vi "niFpgaFFTOutsideSCTLCore.vi"(0 "real data in":fxp<+/-,16,1> format="%#.16g", 1 "reset":bool, 5 "imaginary data in":fxp<+/-,16,1> format="%#.16g") -> (3 "data index":u16, 4 "real data out":fxp<+/-,16,6> format="%.12g", 6 "imaginary data out":fxp<+/-,16,6> format="%.12g", 8 "output valid":bool)   [LabVIEW 2017]
uses:
  <vilib>/rvi/LocalResourceManager/LocalResourceManager.xnode
  <vilib>/rvi/FXPMathLib/basic elements/FxpDiscreteDelay/XNode/nifxpmath_DiscreteDelay.xnode
  <vilib>/Platform/TimedLoop/XDataNode/XDataNode.xnode
  <vilib>/Platform/TimedLoop/XDataNode/nitl_modes.ctl
  <vilib>/Platform/TimedLoop/XDataNode/XDNodeRunTimeDep.lvlib
  <vilib>/Platform/TimedLoop/XDataNode/wakeup.ctl
  <vilib>/Platform/TimedLoop/XDataNode/timing_clust.ctl
  <vilib>/rvi/DataTransferAndStorage/Container/XNode/niFpgaContainer.xnode
  <vilib>/rvi/Memory/Memory_Emulation/niFpgaMemoryEmulationRefIn.vi
  <vilib>/rvi/DataTransferAndStorage/Container/Common/niFpgaContainerGetUniqueNameForEmu.vi
  <vilib>/rvi/DataTransferAndStorage/Container/Common/niFpgaContainerSetEmuInfo.vi
  <vilib>/rvi/eio/common/nirviEmuReportErrorAndStop.vi
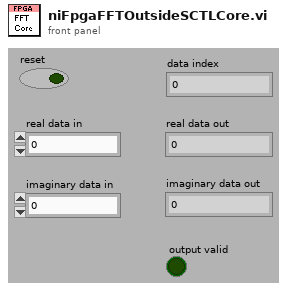
[diagram p1: front panel]
types:
  T1 = typedef "XDNodeRunTimeDep.lvlib/timing_clust.ctl" = cluster{"Expected End [f-1]":u64, "Actual End [f-1]":u64, "Finished Late? [f-1]":bool, "Expected End [i-1]":u64, "Actual End [i-1]":u64, "Finished Late? [i-1]":bool, "Expected Start [i]":u64, "Actual Start [i]":u64, "Expected Start [f]":u64, "Actual Start [f]":u64, "Source Name":string, "Structure Name":string, "Period":i64, "Deadline":i64, "Offset":i64, "Start":i64, "Priority":i32, "Timeout":i32, "Mode":T2, "Wakeup Reason":T3, "Error":errorcluster, "Source Type":string, "Secondary Source Type":string, "Global End Time":u64, "Global Start Time":u64, "Frame Duration":u64, "Iteration Duration":u64, "Assigned CPU":i32, "I/O Scan Engine Mode":u32}
  T2 = typedef "XDNodeRunTimeDep.lvlib/nitl_modes.ctl" = enum32{"No Change", "Process missed periods, maintain original phase", "Discard missed periods, maintain original phase", "Process missed periods, ignore original phase", "Discard missed periods, ignore original phase"}
  T3 = typedef "XDNodeRunTimeDep.lvlib/wakeup.ctl" = enum32{"Normal", "Aborted", "Asynchronous wakeup", "Timing source error", "Timed loop error", "Timeout"}
  T4 = cluster{"N/2-1":u16, "(N/2)*K + 1":u16, "N-1":u16, "total latency":u16, "K - 1":u8, "K - 16":i8, "K - 17":i8}
  T5 = cluster{"Real":fxp<+/-,16,1>, "Imaginary":fxp<+/-,16,1>}
  T6 = typedef "niFPGA FFT Outside SCTL Control Signals.ctl" = cluster{"switch":bool, "twiddle address":u16, "stage":u8, "io read address":u16, "io block 1?":bool, "trans write":bool, "io write address":u16, "update outputs":bool, "use transfer":bool, "io mem a?":bool, "io write":bool, "trans read address":u16}
  T7 = cluster{"addr":u16, "enable":bool, "data":cluster{"Real":fxp<+/-,16,1>, "Imaginary":fxp<+/-,16,1>}}
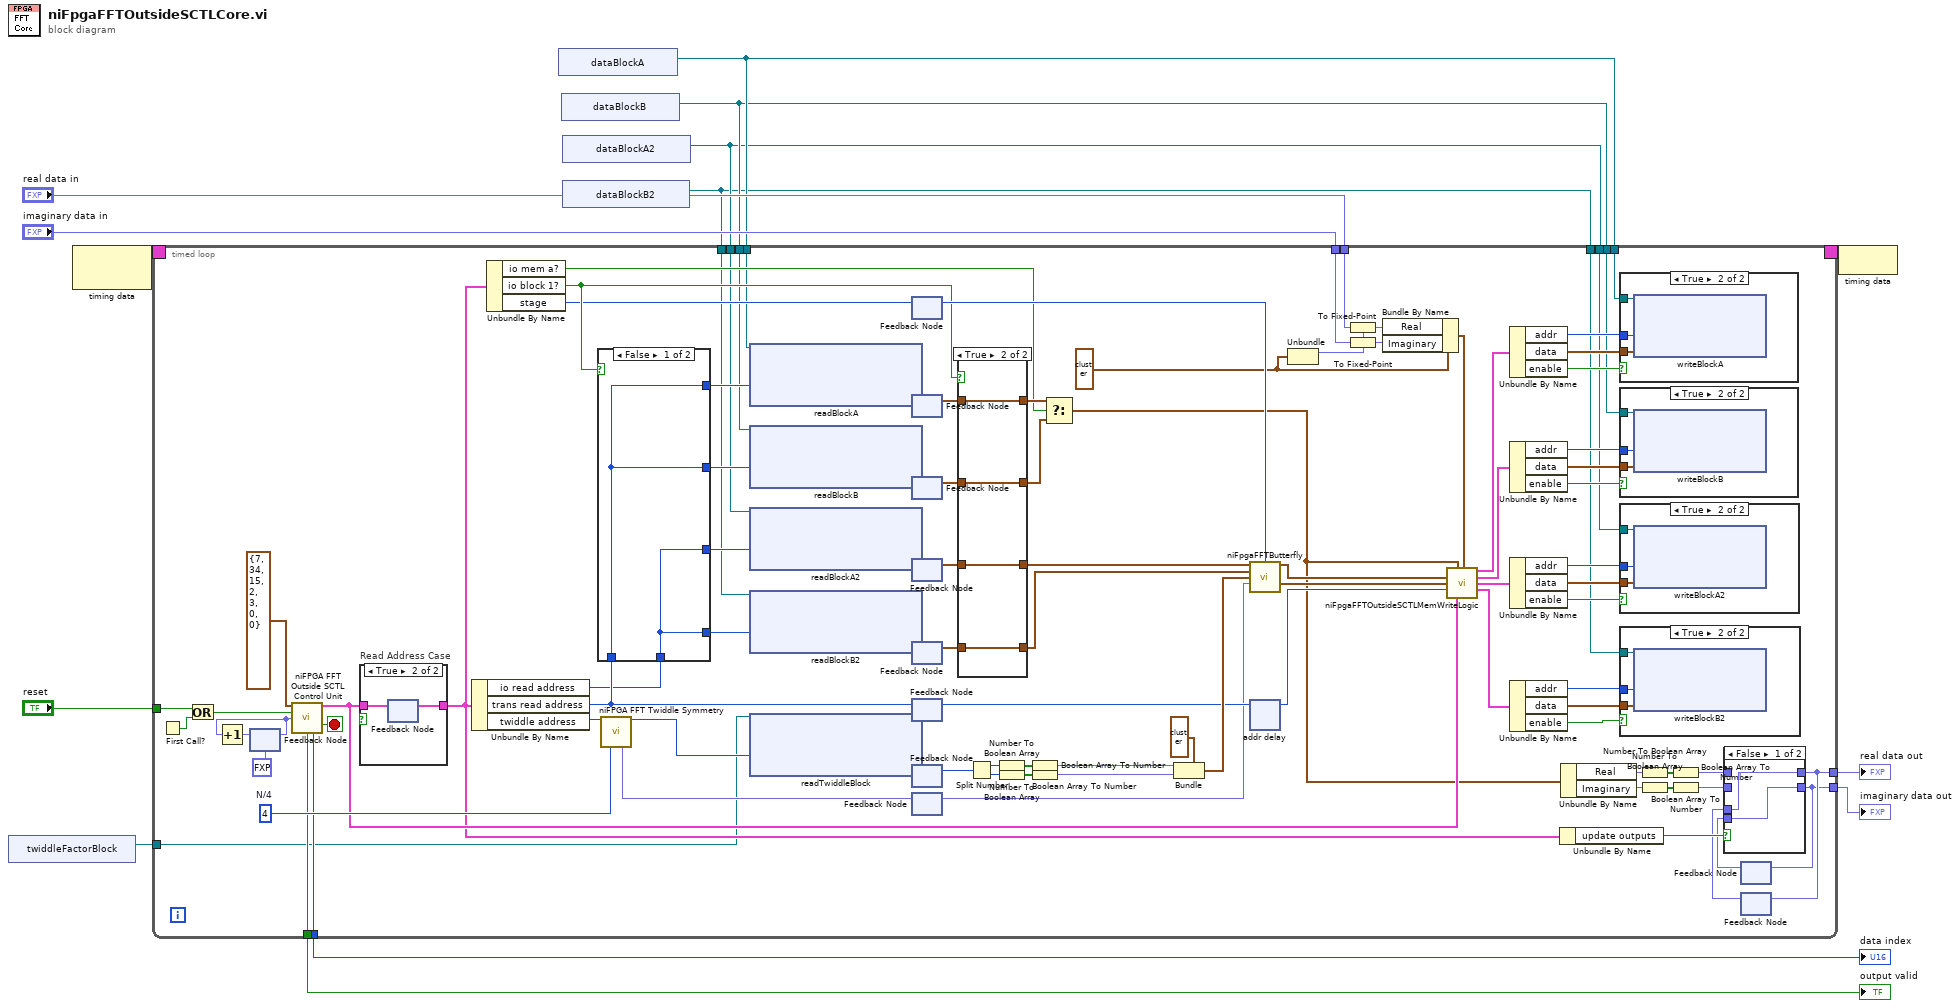
[diagram p0: block diagram]
diagram:
  n1 = xnode "twiddleFactorBlock"() -> ("Memory Out"=w5:refnum<k21>)
  n2 = node-c288() -> (w14:T1)  [unwired: 1 in]
  n3 = xnode "dataBlockA"() -> ("Memory Out"=w4:refnum<k21>)
  n4 = xnode "dataBlockB"() -> ("Memory Out"=w3:refnum<k21>)
  n5 = xnode "dataBlockA2"() -> ("Memory Out"=w2:refnum<k21>)
  n6 = xnode "dataBlockB2"() -> ("Memory Out"=w1:refnum<k21>)
  n7 = timed-loop {
    timing: w14 -> [_]
    timing-out: [_] -> w13
    tunnel: [w53] -> w12
    tunnel: "real data in" -> [w59]
    tunnel: "imaginary data in" -> [w58]
    tunnel: [w55] -> w9
    tunnel: [w54] -> w8
    tunnel: [w52] -> w7
    tunnel: "reset" -> [w30]
    tunnel: w5 -> [w23]
    tunnel: w4 -> [w22]
    tunnel: w3 -> [w21]
    tunnel: w4 -> [w20]
    tunnel: w3 -> [w19]
    tunnel: w2 -> [w18]
    tunnel: w1 -> [w17]
    tunnel: w2 -> [w16]
    tunnel: w1 -> [w15]
    stop <- w50 stop-if-true
    w81 = u16 4  # N/4
    w38 = T5 {"Real"=0.0, "Imaginary"=0.0} ("internalComplexType")
    n8 = First Call?() -> (First Call?: T/F=w32:bool)
    n9 = Or(x=w30, y=w32) -> (x .or. y?=w31:bool)
    n10 = feedback #1(fxp<+,3,3> 0.0) -> (w48:fxp<+,3,3>)
    n11 = Increment(x=w48) -> (x+1=w49:fxp<+,3,3>)
    n12 = feedback-in #1(w49) -> ()
    n13 = call <vilib>:"niFPGA FFT Outside SCTL Control Unit.vi"("Execution Constants"=T4 {"N/2-1"=7, "(N/2)*K + 1"=34, "N-1"=15, "total latency"=2, "K - 1"=3, "K - 16"=0, "K - 17"=0}, "reset"=w31, "iteration"=w48) -> ("control signals out"=w28:T6, "stop"=w50:bool, "output valid"=w52:bool, "data index"=w53:u16)  [unwired: 9 in]
    n14 = case "Read Address Case" shown="True" {
      selector: _ -> [_ _]
      tunnel: w28 -> [w112 w114]
      tunnel: [w112 w113] -> w27
      frame False {
      }
      frame True {
        n15 = feedback-in #2(w114) -> ()
        n16 = feedback #2() -> (w113:T6)  [unwired: 1 in]
      }
    }
    n17 = Unbundle By Name(w27) -> ("io read address"=w64:u16, "trans read address"=w101:u16, "twiddle address"=w33:u16)
    n18 = Unbundle By Name(w27) -> ("io mem a?"=w41:bool, "io block 1?"=w40:bool, "stage"=w29:u8)
    n19 = case shown="False" w40 {
      tunnel: [w127 w130] -> w73
      tunnel: w101 -> [w128 w130]
      tunnel: [w127 w130] -> w72
      tunnel: [w128 w129] -> w71
      tunnel: [w128 w129] -> w70
      tunnel: w64 -> [w127 w129]
      frame False {
      }
      frame True {
      }
    }
    n20 = call <vilib>:"niFPGA FFT Twiddle Symmetry.vi"("twiddle index"=w33, "N/4"=w81) -> ("modified twiddle index"=w37:u16, "flag"=w36:fxp<+,2,2>)  [unwired: 12 in]
    n21 = xnode ("readBlockA")("Address"=w71, "Memory In"=w22) -> ("Data"=w45:T5)  [unwired: 1 out]
    n22 = xnode ("readBlockB")("Address"=w70, "Memory In"=w21) -> ("Data"=w42:T5)  [unwired: 1 out]
    n23 = xnode ("readBlockA2")("Address"=w72, "Memory In"=w18) -> ("Data"=w84:T5)  [unwired: 1 out]
    n24 = xnode ("readBlockB2")("Address"=w73, "Memory In"=w17) -> ("Data"=w83:T5)  [unwired: 1 out]
    n25 = xnode ("readTwiddleBlock")("Address"=w37, "Memory In"=w23) -> ("Data"=w82:u32)  [unwired: 1 out]
    n26 = feedback-in #3(w29) -> ()
    n27 = feedback #3() -> (w46:u8)  [unwired: 1 in]
    n28 = feedback-in #4(w45) -> ()
    n29 = feedback #4() -> (w44:T5)  [unwired: 1 in]
    n30 = feedback-in #5(w42) -> ()
    n31 = feedback #5() -> (w43:T5)  [unwired: 1 in]
    n32 = feedback-in #6(w84) -> ()
    n33 = feedback #6() -> (w63:T5)  [unwired: 1 in]
    n34 = feedback-in #7(w83) -> ()
    n35 = feedback #7() -> (w62:T5)  [unwired: 1 in]
    n36 = feedback-in #8(w101) -> ()
    n37 = feedback #8() -> (w61:u16)  [unwired: 1 in]
    n38 = feedback-in #9(w82) -> ()
    n39 = feedback #9() -> (w60:u32)  [unwired: 1 in]
    n40 = feedback-in #10(w36) -> ()
    n41 = feedback #10() -> (w34:fxp<+,2,2>)  [unwired: 1 in]
    n42 = case shown="True" w40 {
      tunnel: [w119 w126] -> w24
      tunnel: w62 -> [w121 w126]
      tunnel: [w120 w125] -> w25
      tunnel: w63 -> [w122 w125]
      tunnel: [w121 w124] -> w68
      tunnel: w43 -> [w119 w124]
      tunnel: [w122 w123] -> w69
      tunnel: w44 -> [w120 w123]
      frame False {
      }
      frame True {
      }
    }
    n43 = Split Number(x=w60) -> (hi(x)=w74:u16, lo(x)=w77:u16)
    n44 = Number To Boolean Array(number=w74) -> (Boolean array=w80:bool[])
    n45 = Number To Boolean Array(number=w77) -> (Boolean array=w79:bool[])
    n46 = Boolean Array To Number ("fxpForCluster7")(Boolean array=w80) -> (number=w35:fxp<+/-,16,1>)
    n47 = Boolean Array To Number ("fxpForCluster8")(Boolean array=w79) -> (number=w78:fxp<+/-,16,1>)
    n48 = Select(t=w69, s=w41, f=w68) -> (s? t:f=w26:T5)
    n49 = Bundle(cluster=T5 {"Real"=0.0, "Imaginary"=0.0} ("internalTwiddleType"), "Real"=w35, "Imaginary"=w78) -> (w76:T5)
    n50 = call <vilib>:"niFpgaFFTButterfly.vi"("X in"=w25, "stage"=w46, "Y in"=w24, "TwiddleFactor"=w76, "flag"=w34) -> ("X out"=w99:T5, "Y out"=w100:T5)  [unwired: 9 in]
    n51 = xnode ("addr delay")("D"=w61) -> ("Q"=w102:u16)
    n52 = Unbundle(w38) -> ("Real"=w39:fxp<+/-,16,1>)  [unwired: 1 out]
    n53 = To Fixed-Point(fixed-point type=w39, number=w59) -> (fixed-point=w93:fxp<+/-,16,1>)
    n54 = To Fixed-Point(fixed-point type=w39, number=w58) -> (fixed-point=w94:fxp<+/-,16,1>)
    n55 = Bundle By Name(cluster=w38, "Real"=w93, "Imaginary"=w94) -> (w108:T5)
    n56 = call <vilib>:"niFpgaFFTOutsideSCTLMemWriteLogic.vi"("input data"=w108, "transfer data"=w26, "x from bf"=w99, "y from bf"=w100, "read address"=w102, "control signals"=w28) -> ("memory output A"=w104:T7, "memory output B"=w103:T7, "memory output A 2"=w88:T7, "memory output B 2"=w87:T7)  [unwired: 6 in]
    n57 = Unbundle By Name(w104) -> ("addr"=w105:u16, "data"=w106:T5, "enable"=w107:bool)
    n58 = Unbundle By Name(w103) -> ("addr"=w111:u16, "data"=w110:T5, "enable"=w109:bool)
    n59 = Unbundle By Name(w88) -> ("addr"=w91:u16, "data"=w92:T5, "enable"=w85:bool)
    n60 = Unbundle By Name(w87) -> ("addr"=w90:u16, "data"=w89:T5, "enable"=w86:bool)
    n61 = Unbundle By Name(w27) -> ("update outputs"=w65:bool)
    n62 = Unbundle By Name(w26) -> ("Real"=w96:fxp<+/-,16,1>, "Imaginary"=w95:fxp<+/-,16,1>)
    n63 = case shown="True" w107 {
      tunnel: w106 -> [_ w139]
      tunnel: w105 -> [_ w138]
      tunnel: w20 -> [_ w137]
      frame False {
      }
      frame True {
        n64 = xnode ("writeBlockA")("Address"=w138, "Data"=w139, "Memory In"=w137) -> ()  [unwired: 1 in, 2 out]
      }
    }
    n65 = case shown="True" w109 {
      tunnel: w111 -> [_ w142]
      tunnel: w110 -> [_ w141]
      tunnel: w19 -> [_ w140]
      frame False {
      }
      frame True {
        n66 = xnode ("writeBlockB")("Address"=w142, "Data"=w141, "Memory In"=w140) -> ()  [unwired: 1 out]
      }
    }
    n67 = case shown="True" w85 {
      tunnel: w91 -> [_ w135]
      tunnel: w92 -> [_ w136]
      tunnel: w16 -> [_ w134]
      frame False {
      }
      frame True {
        n68 = xnode ("writeBlockA2")("Address"=w135, "Data"=w136, "Memory In"=w134) -> ()  [unwired: 1 out]
      }
    }
    n69 = case shown="True" w86 {
      tunnel: w90 -> [_ w133]
      tunnel: w89 -> [_ w132]
      tunnel: w15 -> [_ w131]
      frame False {
      }
      frame True {
        n70 = xnode ("writeBlockB2")("Address"=w133, "Data"=w132, "Memory In"=w131) -> ()  [unwired: 1 out]
      }
    }
    n71 = Number To Boolean Array(number=w96) -> (Boolean array=w97:bool[])
    n72 = Number To Boolean Array(number=w95) -> (Boolean array=w98:bool[])
    n73 = Boolean Array To Number ("real fxp conv")(Boolean array=w97) -> (number=w66:fxp<+/-,16,6>)
    n74 = Boolean Array To Number ("imag fxp conv")(Boolean array=w98) -> (number=w67:fxp<+/-,16,6>)
    n75 = feedback #11() -> (w57:fxp<+/-,16,6>)  [unwired: 1 in]
    n76 = feedback #12() -> (w56:fxp<+/-,16,6>)  [unwired: 1 in]
    n77 = case shown="False" w65 {
      tunnel: [w115 w118] -> w54
      tunnel: w67 -> [_ w118]
      tunnel: w66 -> [_ w117]
      tunnel: [w116 w117] -> w55
      tunnel: w56 -> [w116 _]
      tunnel: w57 -> [w115 _]
      frame False {
      }
      frame True {
      }
    }
    n78 = feedback-in #11(w54) -> ()
    n79 = feedback-in #12(w55) -> ()
  }
  "output valid" <- w7
  "data index" <- w12
  "real data out" <- w9
  "imaginary data out" <- w8
  n80 = node-c288(w13) -> ()
